vi "Get Current Node Path.vi"(8 "error in (no error)":errorcluster, 11 "Tree Ref":refnum<k24>) -> (0 "error out":errorcluster, 3 "Current Node Path":string)   [LabVIEW 2016, in "System Mapping Tool.lvlib"]
uses:
  System Mapping Tool.lvlib
  NationalInstruments.VeriStand.SystemStorageUI
  NationalInstruments.VeriStand.SystemStorage
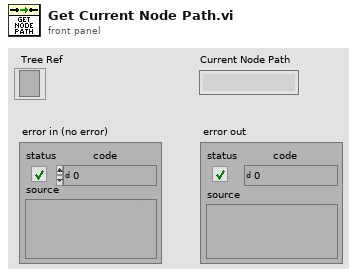
[diagram p1: front panel]
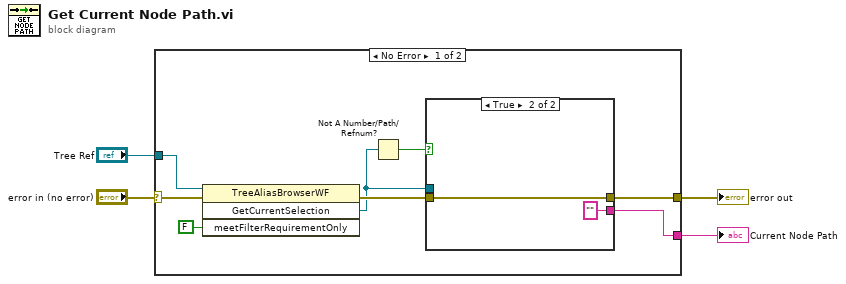
[diagram p0: block diagram]
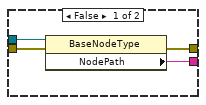
[diagram p2: hidden frame]
diagram:
  n1 = case shown="No Error" "error in (no error)" {
    selector: "error in (no error)" -> [w12 w19]
    tunnel: [w8 w19] -> w3
    tunnel: "Tree Ref" -> [w11 _]
    tunnel: [w7 _] -> w1
    frame No Error {
      n2 = invoke class="TreeAliasBrowserWF" method="GetCurrentSelection"(reference=w11, error in=w12, "meetFilterRequirementOnly"=FALSE) -> (error out=w9:errorcluster, "GetCurrentSelection"=w6:refnum<k24>)  [unwired: 1 in, 2 out]
      n3 = Not A Number/Path/Refnum?(number/path/refnum=w6) -> (NaN/Path/Refnum?=w5:bool)
      n4 = case shown="True" w5 {
        tunnel: w9 -> [w16 w17]
        tunnel: [w15 w17] -> w8
        tunnel: [w14 "" ("NodePath")] -> w7
        tunnel: w6 -> [w13 _]
        frame False {
          n5 = property class="BaseNodeType"(reference=w13, error in=w16) -> (error out=w15:errorcluster, "NodePath"=w14:string)  [unwired: 1 out]
        }
        frame True {
        }
      }
    }
    frame Error {
    }
  }
  "error out" <- w3
  "Current Node Path" <- w1
